vi "Write Solution Table.vi"(8 "Error In":errorcluster, 10 "Layer Information Array":T1 {"Deposition Method" items=["Front Electrode", "Electron Transport Layer", "Active Layer", "Hole Transport Layer", "Back Electrode", "Custom Layer"]; "Layer Type" items=["Front Electrode", "Electron Transport Layer", "Active Layer", "Hole Transport Layer", "Back Electrode", "Custom Layer"]}, 11 "Database Full Information In":T2 {"Database Write Information"."Layer Information Array"."Deposition Method" items=["Blade Coating", "Spin Coating", "Thermal Evaporation", "E-Beam Evaporation", "Sputtering", "Drop Casting", "Dip Coating", "Pulsed Laser Deposition", "Chemival Vapour Deposition", "Atomic Layer Deposition", "Spray Coating", "Screen Printing", "Electroplating", "Molecular Beam Epitaxy", "Custom Deposition"]; "Database Write Information"."Layer Information Array"."Layer Type" items=["Front Electrode", "Electron Transport Layer", "Active Layer", "Hole Transport Layer", "Back Electrode", "Custom Layer"]}) -> (0 "Error Out":errorcluster, 3 "Database Full Information Out":T2 {"Database Write Information"."Layer Information Array"."Deposition Method" items=["Blade Coating", "Spin Coating", "Thermal Evaporation", "E-Beam Evaporation", "Sputtering", "Drop Casting", "Dip Coating", "Pulsed Laser Deposition", "Chemival Vapour Deposition", "Atomic Layer Deposition", "Spray Coating", "Screen Printing", "Electroplating", "Molecular Beam Epitaxy", "Custom Deposition"]; "Database Write Information"."Layer Information Array"."Layer Type" items=["Front Electrode", "Electron Transport Layer", "Active Layer", "Hole Transport Layer", "Back Electrode", "Custom Layer"]})   [LabVIEW 2020]
uses:
  Data Clusters/Database Information.ctl
  Data Clusters/Layer Information Cluster.ctl
  <vilib>/addons/database/Connection.llb/Conn ObjectReference.ctl
  <vilib>/addons/database/NI_Database_API.lvlib
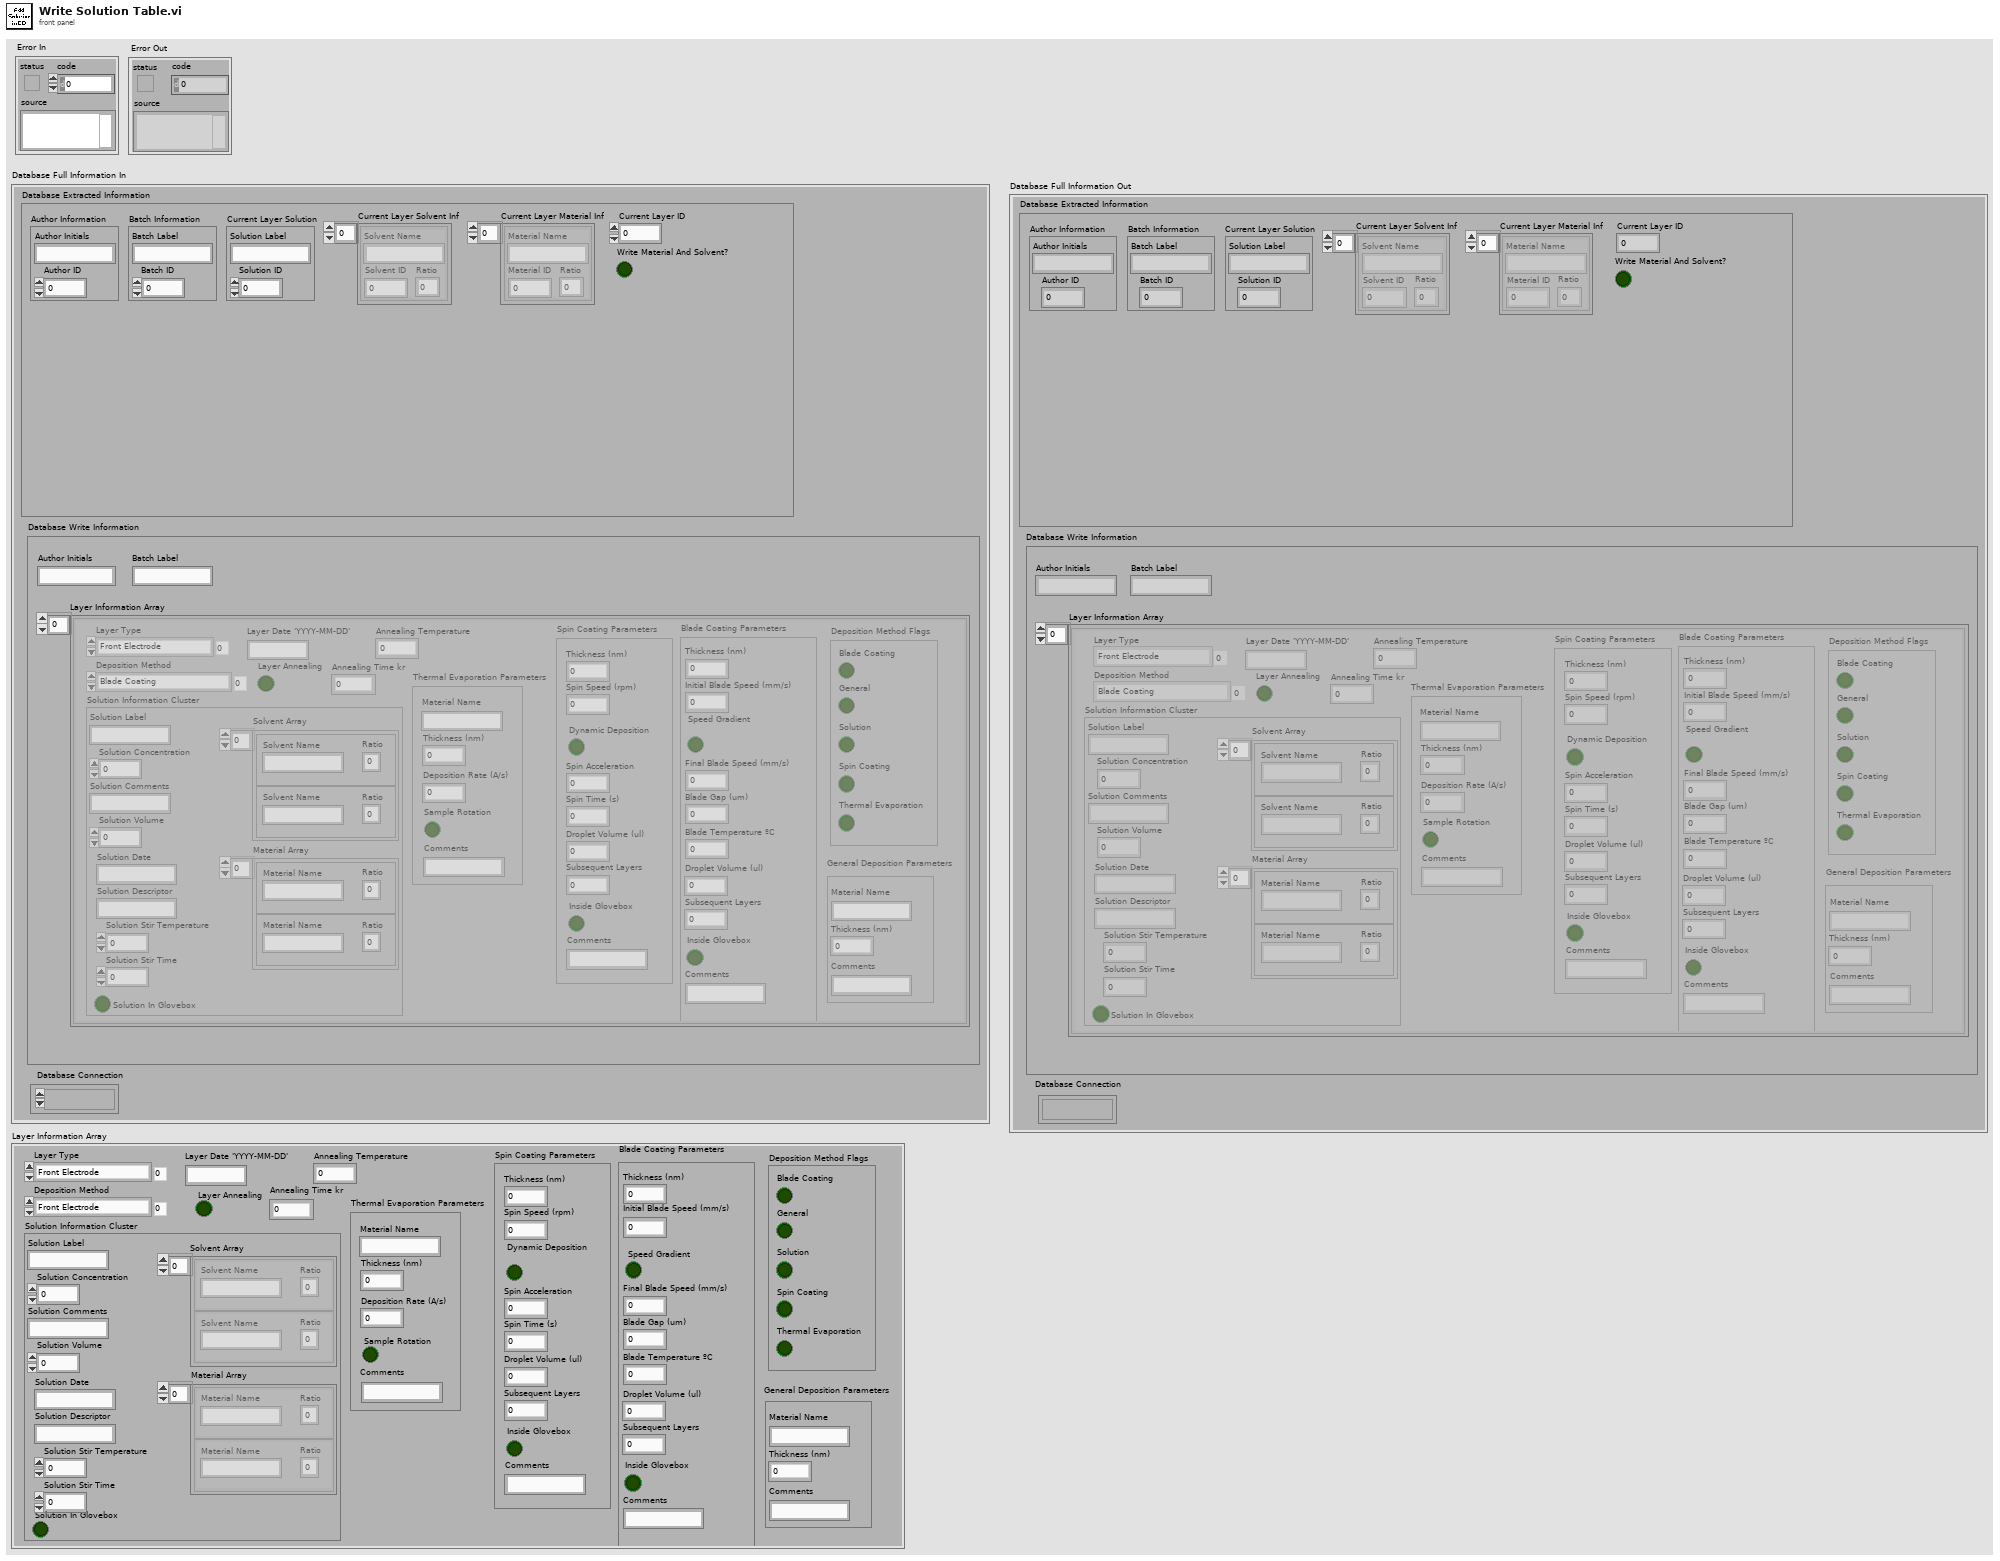
[diagram p1: front panel]
types:
  T1 = typedef "Layer Information Cluster.ctl" = cluster{"Solution Information Cluster":cluster{"Solution Label":string, "Solution Concentration":dbl, "Solution Comments ":string, "Solution Volume ":dbl, "Solution Date ":string, "Solution Descriptor ":string, "Solution Stir Temperature ":dbl, "Solution Stir Time ":dbl, "Solution In Glovebox":bool, "Solvent Array":cluster{"Solvent Name":string, "Ratio":dbl}[], "Material Array":cluster{"Material Name":string, "Ratio":dbl}[]}, "Layer Type":u16, "Deposition Method":u16, "Layer Annealing":bool, "General Deposition Parameters":cluster{"Thickness (nm)":dbl, "Comments":string, "Material Name":string}, "Blade Coating Parameters":cluster{"Thickness (nm)":dbl, "Initial Blade Speed (mm/s)":dbl, "Speed Gradient":bool, "Final Blade Speed (mm/s)":dbl, "Blade Gap (um)":dbl, "Droplet Volume (ul)":dbl, "Subsequent Layers":dbl, "Inside Glovebox":bool, "Comments":string, "Blade Temperature ºC":dbl}, "Spin Coating Parameters":cluster{"Thickness (nm)":dbl, "Spin Speed (rpm)":dbl, "Dynamic Deposition":bool, "Spin Acceleration":dbl, "Spin Time (s)":dbl, "Droplet Volume (ul)":dbl, "Subsequent Layers":dbl, "Inside Glovebox":bool, "Comments":string}, "Thermal Evaporation Parameters":cluster{"Deposition Rate (A/s)":dbl, "Thickness (nm)":dbl, "Comments":string, "Material Name":string, "Sample Rotation":bool}, "Layer Date 'YYYY-MM-DD'":string, "Annealing Time kr":dbl, "Annealing Temperature":dbl, "Deposition Method Flags":cluster{"Blade Coating":bool, "General ":bool, "Solution":bool, "Spin Coating":bool, "Thermal Evaporation":bool}}
  T2 = typedef "Database Information.ctl" = cluster{"Database Extracted Information":cluster{"Author Information":cluster{"Author Initials":string, "Author ID":i32}, "Batch Information":cluster{"Batch Label":string, "Batch ID":i32}, "Current Layer Solution":cluster{"Solution Label":string, "Solution ID":i32}, "Current Layer ID":i32, "Current Layer Solvent Inf":cluster{"Solvent Name":string, "Solvent ID":i32, "Ratio":dbl}[], "Current Layer Material Inf":cluster{"Material Name":string, "Material ID":i32, "Ratio":dbl}[], "Write Material And Solvent?":bool}, "Database Write Information":cluster{"Author Initials":string, "Batch Label":string, "Layer Information Array":T1[]}, "Database Connection":T3}
  T3 = typedef "NI_Database_API.lvlib/Conn ObjectReference.ctl" = refnum<k1>
  T4 = cluster{"Solution Label":string, "Solution ID":i32}
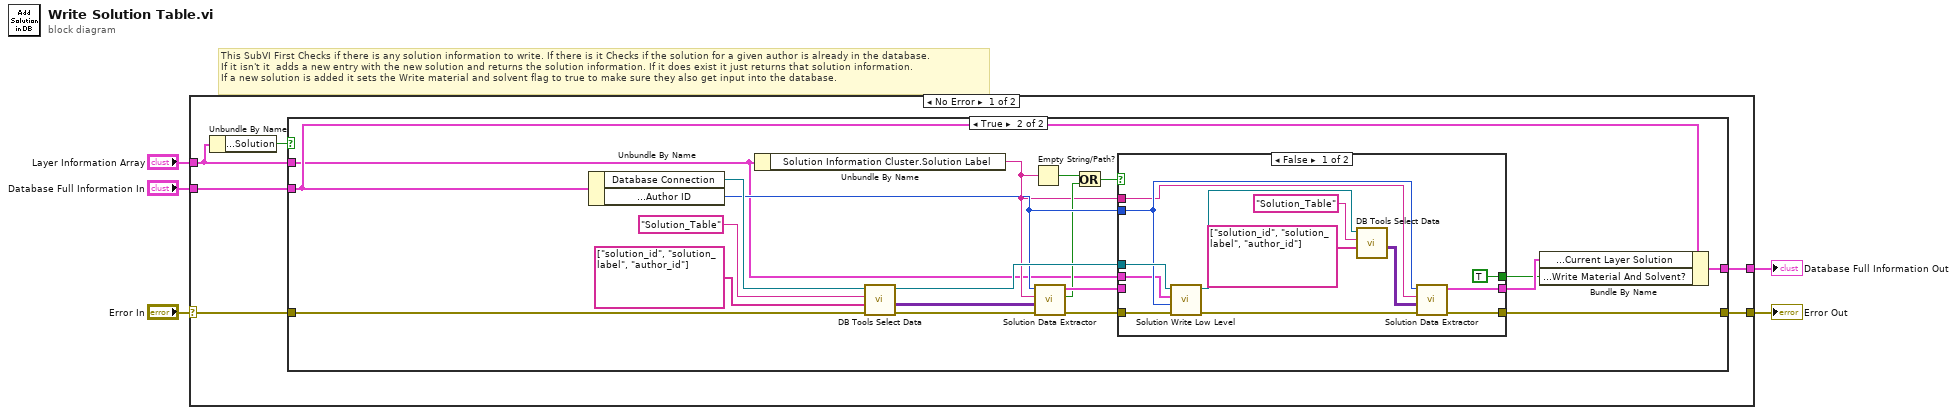
[diagram p0: block diagram]
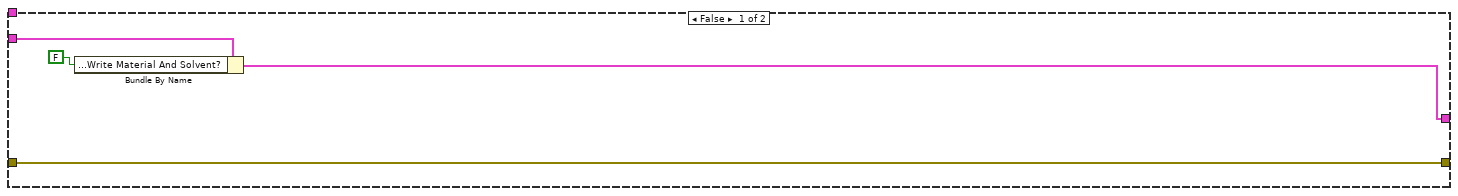
[diagram p2: hidden frame]
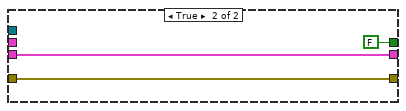
[diagram p3: hidden frame]
diagram:
  # "This SubVI First Checks if there is any solution information to write. If there is it Checks if the solution for a given author is already in the database. \nIf it isn't it  adds a new entry with the new solution and returns the solution information. If it does exist it just returns that solution information.\nIf a new solution is added it sets the Write material and solvent flag to true to make sure they also get input into the database."
  n1 = case shown="No Error" "Error In" {
    selector: "Error In" -> [w11 w53]
    tunnel: [w10 w53] -> w4
    tunnel: "Database Full Information In" -> [w9 w52]
    tunnel: [w8 w52] -> w2
    tunnel: "Layer Information Array" -> [w7 _]
    frame No Error {
      n2 = Unbundle By Name(w7) -> ("Deposition Method Flags.Solution"=w6:bool)
      n3 = case shown="True" w6 {
        tunnel: w11 -> [w15 w32]
        tunnel: [w15 w31] -> w10
        tunnel: w9 -> [w14 w27]
        tunnel: [w13 w26] -> w8
        tunnel: w7 -> [_ w18]
        frame False {
          n4 = Bundle By Name(cluster=w14, "Database Extracted Information.Write Material And Solvent?"=FALSE) -> (w13:T2)
        }
        frame True {
          n5 = Unbundle By Name(w27) -> ("Database Connection"=w28:T3, "Database Extracted Information.Author Information.Author ID"=w23:i32)
          n6 = Unbundle By Name(w18) -> ("Solution Information Cluster.Solution Label"=w19:string)
          n7 = call <vilib>:"DB Tools Select Data.vi"("error in (no error)"=w32, "columns"=string[] ["solution_id", "solution_label", "author_id"], "table"="Solution_Table", "connection reference"=w28) -> ("error out"=w25:errorcluster, "data"=w24:variant[][], "connection reference out"=w35:T3)  [unwired: 2 in]
          n8 = Empty String/Path?(string/path=w19) -> (empty?=w29:bool)
          n9 = call "Solution Data Extractor.vi"("Error In"=w25, "Solution Data"=w24, "Solution Label"=w19, "Author ID"=w23) -> ("Error Out"=w20:errorcluster, "Exists?"=w21:bool, "Solution Information"=w22:T4)  [unwired: 5 in]
          n10 = Or(x=w29, y=w21) -> (x .or. y?=w30:bool)
          n11 = case shown="False" w30 {
            tunnel: w19 -> [w42 _]
            tunnel: w20 -> [w48 w51]
            tunnel: w35 -> [w47 _]
            tunnel: [w38 w51] -> w31
            tunnel: w22 -> [_ w50]
            tunnel: [w39 w50] -> w17
            tunnel: w23 -> [w43 _]
            tunnel: w18 -> [w37 _]
            tunnel: [TRUE FALSE] -> w16
            frame False {
              n12 = call "Solution Write Low Level.vi"("error in (no error)"=w48, "Author ID"=w43, "Layer Information Cluster"=w37, "Database Connection In"=w47) -> ("error out"=w40:errorcluster, "Database Connection Out"=w45:T3)  [unwired: 6 in]
              n13 = call <vilib>:"DB Tools Select Data.vi"("columns"=string[] ["solution_id", "solution_label", "author_id"], "table"="Solution_Table", "connection reference"=w45) -> ("data"=w41:variant[][])  [unwired: 3 in, 2 out]
              n14 = call "Solution Data Extractor.vi"("Error In"=w40, "Solution Data"=w41, "Solution Label"=w42, "Author ID"=w43) -> ("Error Out"=w38:errorcluster, "Solution Information"=w39:T4)  [unwired: 5 in, 1 out]
            }
            frame True {
            }
          }
          n15 = Bundle By Name(cluster=w27, "Database Extracted Information.Current Layer Solution"=w17, "Database Extracted Information.Write Material And Solvent?"=w16) -> (w26:T2)
        }
      }
    }
    frame Error {
    }
  }
  "Error Out" <- w4
  "Database Full Information Out" <- w2
